vi "Build scan patterns.vi"() -> ()   [LabVIEW 2015]
panel:
  out "Array":u16[](array[numeric]) format="%016.0b"
  in  "Enable":bool=TRUE
  out "Port1":u8 format="%.0b"
  out "Port1Bit5":bool
  out "Port1Bit4":bool
  out "Port0":u8 format="%.0b"
  in  "LedScanDebEn":bool
  in  "ActiveLedIndexDeb":u16
  in  "ActiveLedIndex":u16
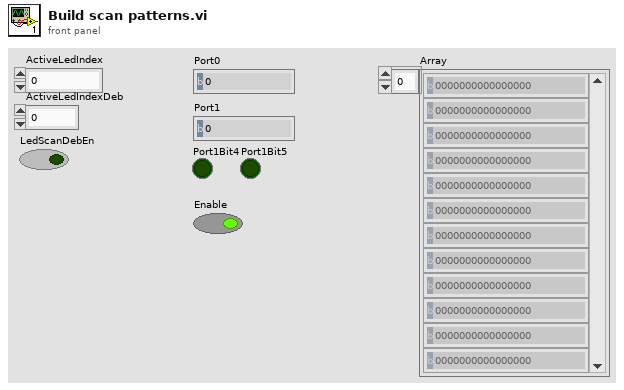
[diagram p1: front panel]
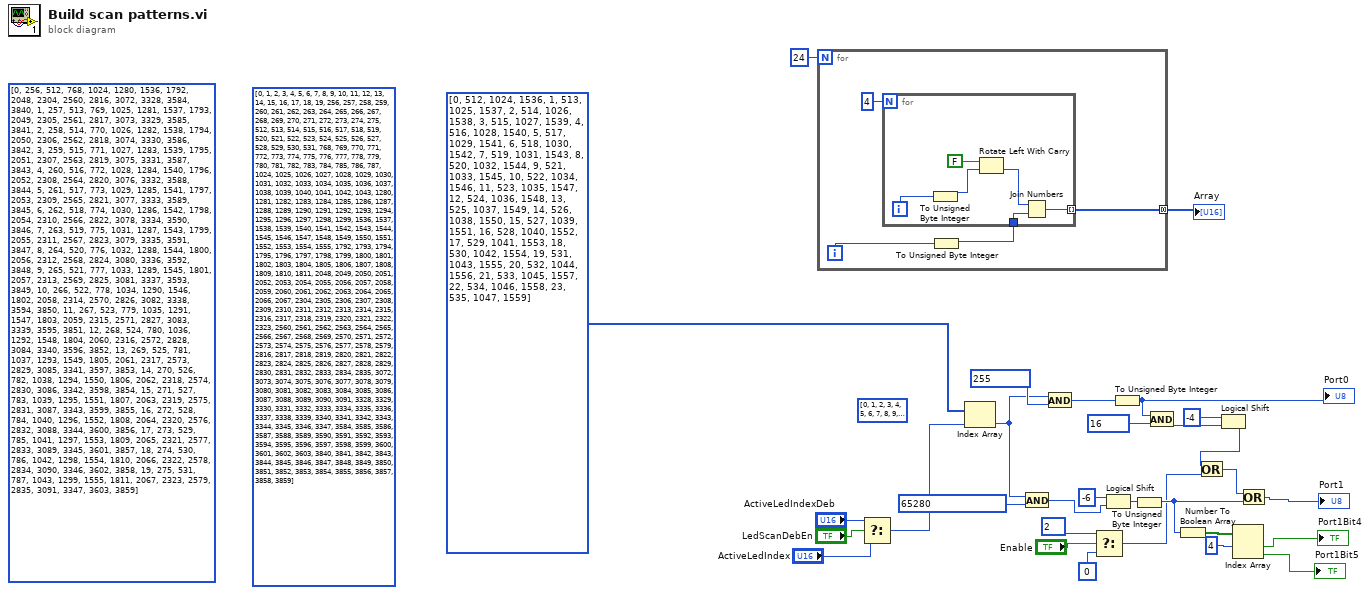
[diagram p0: block diagram]
diagram:
  (unwired) u16[] [0, 256, 512, 768, 1024, 1280, 1536, 1792, 2048, 2304, 2560, 2816, 3072, 3328, 3584, 3840, 1, 257, 513, 769, 1025, 1281, 1537, 1793, 2049, 2305, 2561, 2817, 3073, 3329, 3585, 3841, 2, 258, 514, 770, 1026, 1282, 1538, 1794, 2050, 2306, 2562, 2818, 3074, 3330, 3586, 3842, 3, 259, 515, 771, 1027, 1283, 1539, 1795, 2051, 2307, 2563, 2819, 3075, 3331, 3587, 3843, 4, 260, 516, 772, 1028, 1284, 1540, 1796, 2052, 2308, 2564, 2820, 3076, 3332, 3588, 3844, 5, 261, 517, 773, 1029, 1285, 1541, 1797, 2053, 2309, 2565, 2821, 3077, 3333, 3589, 3845, 6, 262, 518, 774, 1030, 1286, 1542, 1798, 2054, 2310, 2566, 2822, 3078, 3334, 3590, 3846, 7, 263, 519, 775, 1031, 1287, 1543, 1799, 2055, 2311, 2567, 2823, 3079, 3335, 3591, 3847, 8, 264, 520, 776, 1032, 1288, 1544, 1800, 2056, 2312, 2568, 2824, 3080, 3336, 3592, 3848, 9, 265, 521, 777, 1033, 1289, 1545, 1801, 2057, 2313, 2569, 2825, 3081, 3337, 3593, 3849, 10, 266, 522, 778, 1034, 1290, 1546, 1802, 2058, 2314, 2570, 2826, 3082, 3338, 3594, 3850, 11, 267, 523, 779, 1035, 1291, 1547, 1803, 2059, 2315, 2571, 2827, 3083, 3339, 3595, 3851, 12, 268, 524, 780, 1036, 1292, 1548, 1804, 2060, 2316, 2572, 2828, 3084, 3340, 3596, 3852, 13, 269, 525, 781, 1037, 1293, 1549, 1805, 2061, 2317, 2573, 2829, 3085, 3341, 3597, 3853, 14, 270, 526, 782, 1038, 1294, 1550, 1806, 2062, 2318, 2574, 2830, 3086, 3342, 3598, 3854, 15, 271, 527, 783, 1039, 1295, 1551, 1807, 2063, 2319, 2575, 2831, 3087, 3343, 3599, 3855, 16, 272, 528, 784, 1040, 1296, 1552, 1808, 2064, 2320, 2576, 2832, 3088, 3344, 3600, 3856, 17, 273, 529, 785, 1041, 1297, 1553, 1809, 2065, 2321, 2577, 2833, 3089, 3345, 3601, 3857, 18, 274, 530, 786, 1042, 1298, 1554, 1810, 2066, 2322, 2578, 2834, 3090, 3346, 3602, 3858, 19, 275, 531, 787, 1043, 1299, 1555, 1811, 2067, 2323, 2579, 2835, 3091, 3347, 3603, 3859] ("Array")
  (unwired) u16[] [0, 1, 2, 3, 4, 5, 6, 7, 8, 9, 10, 11, 12, 13, 14, 15, 16, 17, 18, 19, 256, 257, 258, 259, 260, 261, 262, 263, 264, 265, 266, 267, 268, 269, 270, 271, 272, 273, 274, 275, 512, 513, 514, 515, 516, 517, 518, 519, 520, 521, 522, 523, 524, 525, 526, 527, 528, 529, 530, 531, 768, 769, 770, 771, 772, 773, 774, 775, 776, 777, 778, 779, 780, 781, 782, 783, 784, 785, 786, 787, 1024, 1025, 1026, 1027, 1028, 1029, 1030, 1031, 1032, 1033, 1034, 1035, 1036, 1037, 1038, 1039, 1040, 1041, 1042, 1043, 1280, 1281, 1282, 1283, 1284, 1285, 1286, 1287, 1288, 1289, 1290, 1291, 1292, 1293, 1294, 1295, 1296, 1297, 1298, 1299, 1536, 1537, 1538, 1539, 1540, 1541, 1542, 1543, 1544, 1545, 1546, 1547, 1548, 1549, 1550, 1551, 1552, 1553, 1554, 1555, 1792, 1793, 1794, 1795, 1796, 1797, 1798, 1799, 1800, 1801, 1802, 1803, 1804, 1805, 1806, 1807, 1808, 1809, 1810, 1811, 2048, 2049, 2050, 2051, 2052, 2053, 2054, 2055, 2056, 2057, 2058, 2059, 2060, 2061, 2062, 2063, 2064, 2065, 2066, 2067, 2304, 2305, 2306, 2307, 2308, 2309, 2310, 2311, 2312, 2313, 2314, 2315, 2316, 2317, 2318, 2319, 2320, 2321, 2322, 2323, 2560, 2561, 2562, 2563, 2564, 2565, 2566, 2567, 2568, 2569, 2570, 2571, 2572, 2573, 2574, 2575, 2576, 2577, 2578, 2579, 2816, 2817, 2818, 2819, 2820, 2821, 2822, 2823, 2824, 2825, 2826, 2827, 2828, 2829, 2830, 2831, 2832, 2833, 2834, 2835, 3072, 3073, 3074, 3075, 3076, 3077, 3078, 3079, 3080, 3081, 3082, 3083, 3084, 3085, 3086, 3087, 3088, 3089, 3090, 3091, 3328, 3329, 3330, 3331, 3332, 3333, 3334, 3335, 3336, 3337, 3338, 3339, 3340, 3341, 3342, 3343, 3344, 3345, 3346, 3347, 3584, 3585, 3586, 3587, 3588, 3589, 3590, 3591, 3592, 3593, 3594, 3595, 3596, 3597, 3598, 3599, 3600, 3601, 3602, 3603, 3840, 3841, 3842, 3843, 3844, 3845, 3846, 3847, 3848, 3849, 3850, 3851, 3852, 3853, 3854, 3855, 3856, 3857, 3858, 3859] ("Array")
  (unwired) u16[] [0, 1, 2, 3, 4, 5, 6, 7, 8, 9, 10, 11, 12, 13, 14, 15, 16, 17, 18, 19, 256, 257, 258, 259, 260, 261, 262, 263, 264, 265, 266, 267, 268, 269, 270, 271, 272, 273, 274, 275, 512, 513, 514, 515, 516, 517, 518, 519, 520, 521, 522, 523, 524, 525, 526, 527, 528, 529, 530, 531, 768, 769, 770, 771, 772, 773, 774, 775, 776, 777, 778, 779, 780, 781, 782, 783, 784, 785, 786, 787, 1024, 1025, 1026, 1027, 1028, 1029, 1030, 1031, 1032, 1033, 1034, 1035, 1036, 1037, 1038, 1039, 1040, 1041, 1042, 1043, 1280, 1281, 1282, 1283, 1284, 1285, 1286, 1287, 1288, 1289, 1290, 1291, 1292, 1293, 1294, 1295, 1296, 1297, 1298, 1299, 1536, 1537, 1538, 1539, 1540, 1541, 1542, 1543, 1544, 1545, 1546, 1547, 1548, 1549, 1550, 1551, 1552, 1553, 1554, 1555, 1792, 1793, 1794, 1795, 1796, 1797, 1798, 1799, 1800, 1801, 1802, 1803, 1804, 1805, 1806, 1807, 1808, 1809, 1810, 1811, 2048, 2049, 2050, 2051, 2052, 2053, 2054, 2055, 2056, 2057, 2058, 2059, 2060, 2061, 2062, 2063, 2064, 2065, 2066, 2067, 2304, 2305, 2306, 2307, 2308, 2309, 2310, 2311, 2312, 2313, 2314, 2315, 2316, 2317, 2318, 2319, 2320, 2321, 2322, 2323, 2560, 2561, 2562, 2563, 2564, 2565, 2566, 2567, 2568, 2569, 2570, 2571, 2572, 2573, 2574, 2575, 2576, 2577, 2578, 2579, 2816, 2817, 2818, 2819, 2820, 2821, 2822, 2823, 2824, 2825, 2826, 2827, 2828, 2829, 2830, 2831, 2832, 2833, 2834, 2835, 3072, 3073, 3074, 3075, 3076, 3077, 3078, 3079, 3080, 3081, 3082, 3083, 3084, 3085, 3086, 3087, 3088, 3089, 3090, 3091, 3328, 3329, 3330, 3331, 3332, 3333, 3334, 3335, 3336, 3337, 3338, 3339, 3340, 3341, 3342, 3343, 3344, 3345, 3346, 3347, 3584, 3585, 3586, 3587, 3588, 3589, 3590, 3591, 3592, 3593, 3594, 3595, 3596, 3597, 3598, 3599, 3600, 3601, 3602, 3603, 3840, 3841, 3842, 3843, 3844, 3845, 3846, 3847, 3848, 3849, 3850, 3851, 3852, 3853, 3854, 3855, 3856, 3857, 3858, 3859] ("Array")
  n1 = for {
    N: 24 -> [_]
    tunnel: [w31] -> w4 mode=concatenating
    i -> [w33]
    n2 = To Unsigned Byte Integer(number=w33) -> (unsigned 8bit integer=w32:u8)
    n3 = for {
      N: 4 -> [_]
      tunnel: w32 -> [w39]
      tunnel: [w38] -> w31 mode=indexing
      i -> [w40]
      n4 = To Unsigned Byte Integer(number=w40) -> (unsigned 8bit integer=w36:u8)
      n5 = Rotate Left With Carry(2:w36, 3:FALSE ("carry")) -> (0:w35:u8)  [unwired: 1 out]
      n6 = Join Numbers(hi=w35, lo=w39) -> ((hi.lo)=w38:u16)
    }
  }
  "Array" <- w4
  n7 = Select(t="ActiveLedIndexDeb", s="LedScanDebEn", f="ActiveLedIndex") -> (s? t:f=w12:u16)
  n8 = Index Array(array=u16[] [0, 512, 1024, 1536, 1, 513, 1025, 1537, 2, 514, 1026, 1538, 3, 515, 1027, 1539, 4, 516, 1028, 1540, 5, 517, 1029, 1541, 6, 518, 1030, 1542, 7, 519, 1031, 1543, 8, 520, 1032, 1544, 9, 521, 1033, 1545, 10, 522, 1034, 1546, 11, 523, 1035, 1547, 12, 524, 1036, 1548, 13, 525, 1037, 1549, 14, 526, 1038, 1550, 15, 527, 1039, 1551, 16, 528, 1040, 1552, 17, 529, 1041, 1553, 18, 530, 1042, 1554, 19, 531, 1043, 1555, 20, 532, 1044, 1556, 21, 533, 1045, 1557, 22, 534, 1046, 1558, 23, 535, 1047, 1559] ("Array"), index=w12) -> (element=w24:u16)
  n9 = And(x=w24, y=u16 65280) -> (x .and. y?=w21:u16)
  n10 = And(x=w24, y=u16 255) -> (x .and. y?=w22:u16)
  n11 = Select(t=u8 2, s="Enable", f=u8 0) -> (s? t:f=w8:u8)
  n12 = Logical Shift(y=i16 -6, x=w21) -> (x << y=w20:u16)
  n13 = To Unsigned Byte Integer(number=w22) -> (unsigned 8bit integer=w18:u8)
  "Port0" <- w18
  n14 = To Unsigned Byte Integer(number=w20) -> (unsigned 8bit integer=w14:u8)
  n15 = And(x=w18, y=u8 16) -> (x .and. y?=w17:u8)
  n16 = Number To Boolean Array(number=w14) -> (Boolean array=w30:bool[])
  n17 = Logical Shift(y=i16 -4, x=w17) -> (x << y=w11:u8)
  n18 = Or(x=w11, y=w8) -> (x .or. y?=w7:u8)
  n19 = Index Array(array=w30, index #1=4 ("index")) -> (element #1=→"Port1Bit4":bool, element #2=→"Port1Bit5":bool)  [unwired: 1 in]
  n20 = Or(x=w7, y=w14) -> (x .or. y?=→"Port1":u8)
